vi "Day03-1.vi"() -> ()   [LabVIEW 2021]
panel:
  out "power":u32
  out "epsilon":u32
  out "gamma":u32
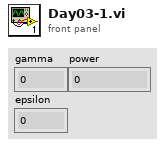
[diagram p1: front panel]
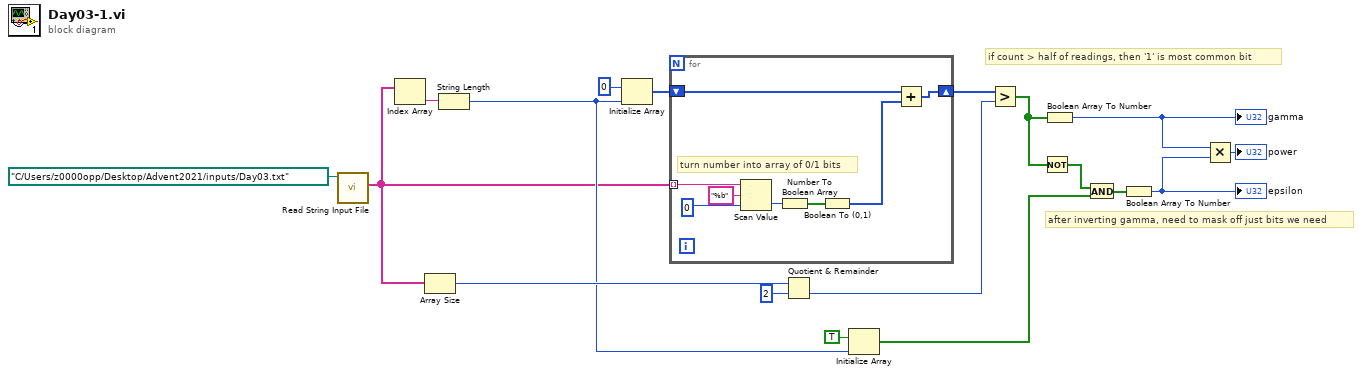
[diagram p0: block diagram]
diagram:
  # "after inverting gamma, need to mask off just bits we need"
  # "if count > half of readings, then '1' is most common bit"
  n1 = call "Read String Input File.vi"("file path (dialog if empty)"=path "C:/Users/z0000opp/Desktop/Advent2021/inputs/Day03.txt") -> ("input values"=w2:string[])  [unwired: 10 in]
  n2 = Index Array(array=w2) -> (element=w6:string)  [unwired: 1 in]
  n3 = Array Size(array=w2) -> (size(s)=w7:i32)
  n4 = String Length(string=w6) -> (length=w5:i32)
  n5 = Initialize Array(i16 0, w5) -> (w18:i16[])
  n6 = for {
    tunnel: w2 -> [w26] mode=indexing
    shift-right: [w20] -> w16
    shift-left: w18 -> [w19]
    # "turn number into array of 0/1 bits"
    n7 = Scan Value(string=w26, format string="%b", default (0 dbl)=u16 0) -> (value=w23:u16)  [unwired: 1 out]
    n8 = Number To Boolean Array(number=w23) -> (Boolean array=w22:bool[])
    n9 = Boolean To (0,1)(Boolean=w22) -> (0, 1=w21:i16[])
    n10 = Add(x=w19, y=w21) -> (x+y=w20:i16[])
  }
  n11 = Quotient & Remainder(x=w7, y=2) -> (floor(x/y)=w15:i32)  [unwired: 1 out]
  n12 = Initialize Array(TRUE, w5) -> (w3:bool[])
  n13 = Greater?(x=w16, y=w15) -> (0:w13:bool[])
  n14 = Not(x=w13) -> (.not. x?=w12:bool[])
  n15 = Boolean Array To Number(Boolean array=w13) -> (number=w9:u32)
  "gamma" <- w9
  n16 = And(x=w12, y=w3) -> (x .and. y?=w11:bool[])
  n17 = Boolean Array To Number(Boolean array=w11) -> (number=w10:u32)
  "epsilon" <- w10
  n18 = Multiply(x=w9, y=w10) -> (x*y=→"power":u32)
